vi "Handle Selection on Ctrl Key.vi"(7 "Ctrl":bool, 8 "error in (no error)":errorcluster, 9 "Shape in":refnum<data-value>[](array[refnum]), 10 "Selected in":i16[](array[numeric]), 11 "Image in":refnum<class "Image.lvclass">) -> (0 "error out":errorcluster, 1 "Shape out":refnum<data-value>[](array[refnum]), 2 "Selected out":i16[](array[numeric]), 3 "Image out":refnum<class "Image.lvclass">)   [LabVIEW 2015, in "LV Image Editor Framework.lvlib" / "Image Editor Handler.lvclass"]
uses:
  Image Editor Handler.lvclass
  Image/Image.lvclass
  Forms/Shape/Shape.lvclass
  Forms/Selection/Selection.lvclass
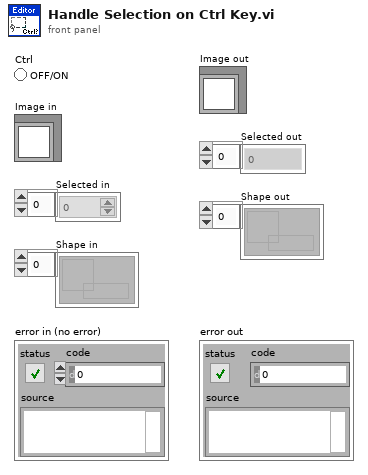
[diagram p1: front panel]
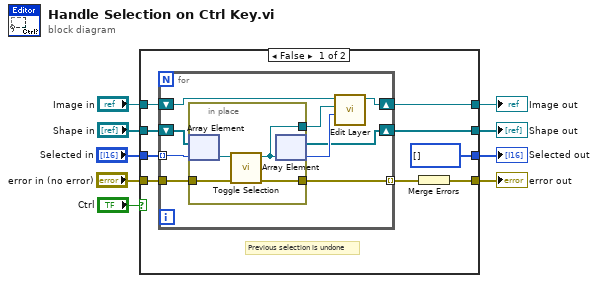
[diagram p0: block diagram]
diagram:
  n1 = case shown="False" "Ctrl" {
    tunnel: [i16[] [] ("Selected") w35] -> w2
    tunnel: "Selected in" -> [w17 w35]
    tunnel: "Shape in" -> [w16 w34]
    tunnel: [w13 w34] -> w5
    tunnel: "Image in" -> [w15 w33]
    tunnel: [w14 w33] -> w7
    tunnel: [w11 w32] -> w8
    tunnel: "error in (no error)" -> [w10 w32]
    frame False {
      # "Previous selection is undone"
      n2 = for {
        shift-right: [w21] -> w14
        shift-left: w15 -> [w22]
        tunnel: w17 -> [w26] mode=indexing
        shift-right: [w23] -> w13
        shift-left: w16 -> [w27]
        tunnel: [w20] -> w12 mode=indexing
        tunnel: w10 -> [w19]
        n3 = in-place {
          in-place-border: [w30] -> w24
          in-place-border: [w29] -> w20
          in-place-border: w19 -> [w28]
          n4 = in-place-array #1(w27, w26) -> (w31:refnum<data-value>)
          n5 = call "Toggle Selection.vi"("error in (no error)"=w28, "Shape"=w31) -> ("error out"=w29:errorcluster, "Shape"=w30:refnum<data-value>)  [unwired: 7 in, 1 out]
          n6 = in-place-array #1(w30) -> (w23:refnum<data-value>[], w25:i32)
        }
        n7 = call "Edit Layer.vi"("Layer Index"=w25, "ShapeRef"=w24, "Image in"=w22) -> ("Image out"=w21:refnum<class "Image.lvclass">)  [unwired: 7 in, 1 out]
      }
      n8 = Merge Errors(w12) -> (w11:errorcluster)
    }
    frame True {
      # "Ctrl enabled => We don't erase the previous selection"
    }
  }
  "error out" <- w8
  "Image out" <- w7
  "Shape out" <- w5
  "Selected out" <- w2
